vi "Create CI Frequency Channel Wrapper.vi"(0 "Task map in":map{string, refnum<k21>}(c390), 5 "Message Data in":T2, 11 "error in (no error)":errorcluster) -> (4 "Task map out":map{string, refnum<k21>}(c390), 6 "Message Data out":T1, 15 "error out":errorcluster)   [LabVIEW 2021, in "NI DAQmx_wrapper.lvlib"]
uses:
  NI DAQmx_wrapper.lvlib
  NI DAQmx_server/RPC Messages/nidaqmx_grpc_CreateCIFreqChanRequest.ctl
  NI DAQmx_server/RPC Messages/nidevice_grpc_Session_session/nidevice_grpc_Session_session.lvclass
  NI DAQmx_server/RPC Messages/nidaqmx_grpc_CreateCIFreqChanRequest_units_enum/nidaqmx_grpc_CreateCIFreqChanRequest_units_enum.lvclass
  NI DAQmx_server/RPC Messages/nidaqmx_grpc_CreateCIFreqChanRequest_edge_enum/nidaqmx_grpc_CreateCIFreqChanRequest_edge_enum.lvclass
  NI DAQmx_server/RPC Messages/nidaqmx_grpc_CreateCIFreqChanRequest_meas_method_enum/nidaqmx_grpc_CreateCIFreqChanRequest_meas_method_enum.lvclass
  NI DAQmx_server/RPC Messages/nidevice_grpc_Session.ctl
  NI DAQmx_server/RPC Messages/nidaqmx_grpc_CreateCIFreqChanResponse.ctl
  NI DAQmx_server/RPC Messages/nidaqmx_grpc_CreateCIFreqChanRequest_edge_enum/nidaqmx_grpc_CreateCIFreqChanRequest_edge_enum.lvclass/nidaqmx_grpc_CreateCIFreqChanRequest_edge_enum.ctl
  NI DAQmx_server/RPC Messages/nidaqmx_grpc_CreateCIFreqChanRequest_units_enum/nidaqmx_grpc_CreateCIFreqChanRequest_units_enum.lvclass/nidaqmx_grpc_CreateCIFreqChanRequest_units_enum.ctl
  NI DAQmx_server/RPC Messages/nidaqmx_grpc_CreateCIFreqChanRequest_meas_method_enum/nidaqmx_grpc_CreateCIFreqChanRequest_meas_method_enum.lvclass/nidaqmx_grpc_CreateCIFreqChanRequest_meas_method_enum.ctl
  NI DAQmx_server/RPC Messages/nidevice_grpc_Session_session/nidevice_grpc_Session_session.lvclass/nidevice_grpc_Session_session.ctl
  <vilib>/DAQmx/create/channels.llb/DAQmx Create Channel (CI-Frequency).vi
  NI DAQmx_server/NI DAQmx_server.lvlib
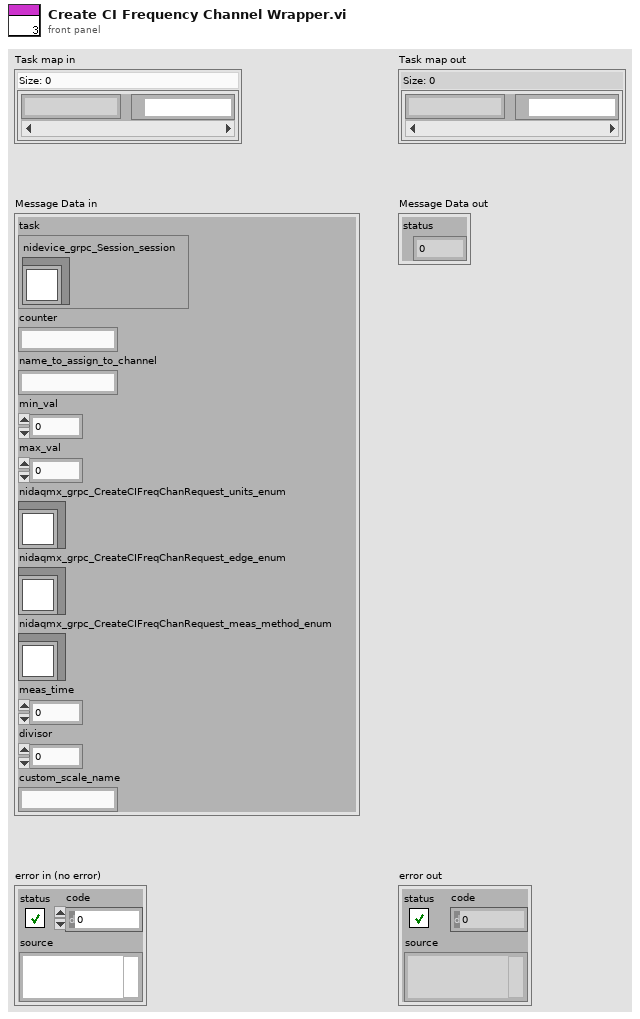
[diagram p1: front panel]
types:
  T1 = typedef "NI DAQmx_server.lvlib/nidaqmx_grpc_CreateCIFreqChanResponse.ctl" = cluster{"status":i32}
  T2 = typedef "NI DAQmx_server.lvlib/nidaqmx_grpc_CreateCIFreqChanRequest.ctl" = cluster{"task":T3, "counter":string, "name_to_assign_to_channel":string, "min_val":dbl, "max_val":dbl, "nidaqmx_grpc_CreateCIFreqChanRequest_units_enum":refnum<class "nidaqmx_grpc_CreateCIFreqChanRequest_units_enum.lvclass">, "nidaqmx_grpc_CreateCIFreqChanRequest_edge_enum":refnum<class "nidaqmx_grpc_CreateCIFreqChanRequest_edge_enum.lvclass">, "nidaqmx_grpc_CreateCIFreqChanRequest_meas_method_enum":refnum<class "nidaqmx_grpc_CreateCIFreqChanRequest_meas_method_enum.lvclass">, "meas_time":dbl, "divisor":u32, "custom_scale_name":string}
  T3 = typedef "NI DAQmx_server.lvlib/nidevice_grpc_Session.ctl" = cluster{"nidevice_grpc_Session_session":refnum<class "nidevice_grpc_Session_session.lvclass">}
  T4 = typedef "NI DAQmx_server.lvlib/nidaqmx_grpc_Edge1.ctl" = enum32{"EDGE1_UNSPECIFIED", "EDGE1_RISING", "EDGE1_FALLING"}
  T5 = typedef "NI DAQmx_server.lvlib/nidaqmx_grpc_FrequencyUnits3.ctl" = enum32{"FREQUENCY_UNITS3_UNSPECIFIED", "FREQUENCY_UNITS3_HZ", "FREQUENCY_UNITS3_TICKS", "FREQUENCY_UNITS3_FROM_CUSTOM_SCALE"}
  T6 = typedef "NI DAQmx_server.lvlib/nidaqmx_grpc_CounterFrequencyMethod.ctl" = enum32{"COUNTER_FREQUENCY_METHOD_UNSPECIFIED", "COUNTER_FREQUENCY_METHOD_LOW_FREQ_1_CTR", "COUNTER_FREQUENCY_METHOD_HIGH_FREQ_2_CTR", "COUNTER_FREQUENCY_METHOD_LARGE_RNG_2_CTR", "COUNTER_FREQUENCY_METHOD_DYN_AVG"}
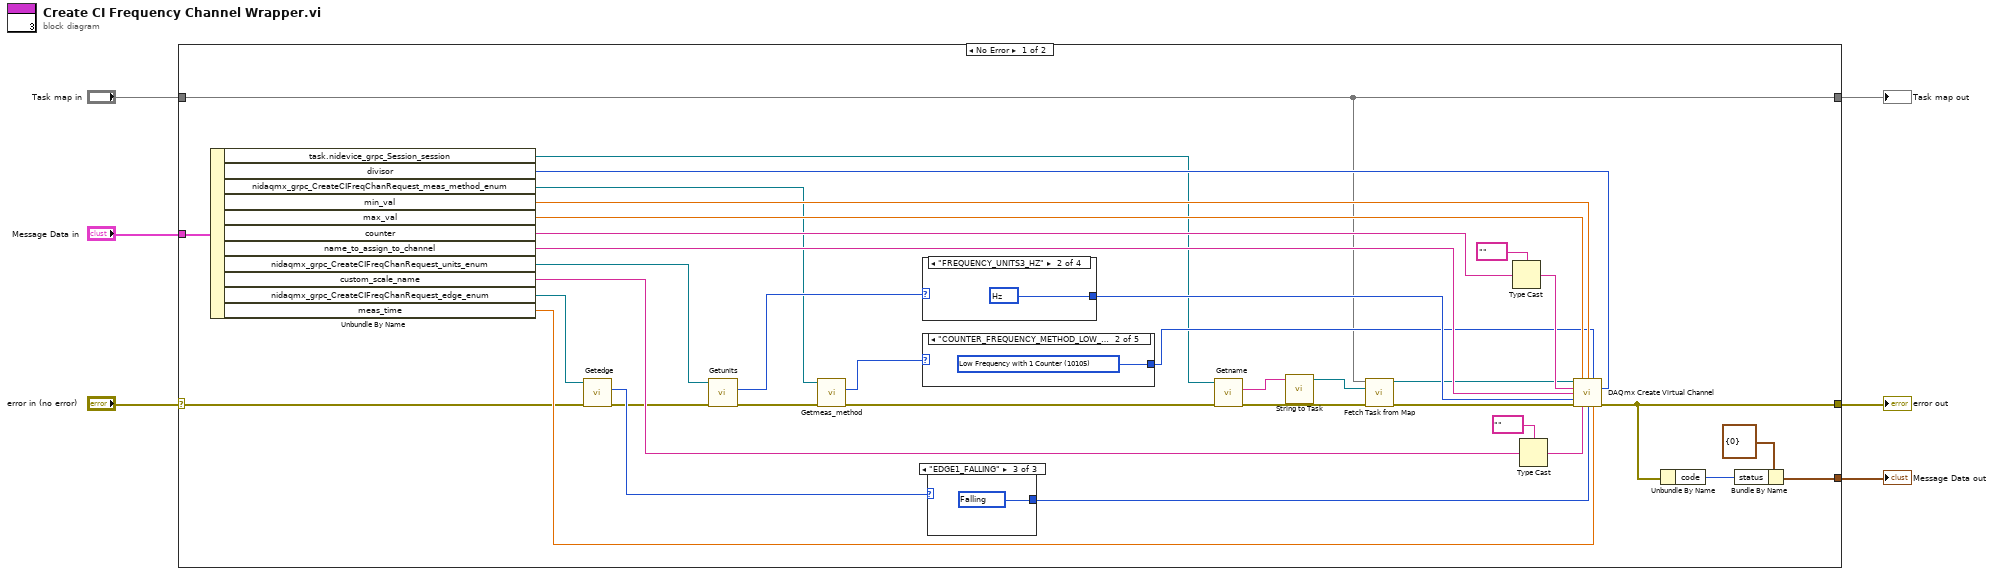
[diagram p0: block diagram]
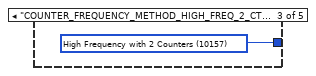
[diagram p3: hidden frame]
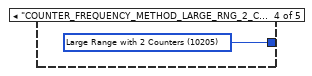
[diagram p4: hidden frame]
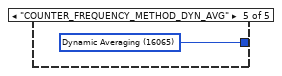
[diagram p5: hidden frame]
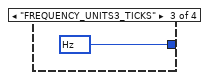
[diagram p7: hidden frame]
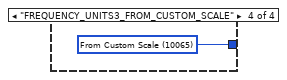
[diagram p8: hidden frame]
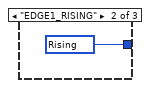
[diagram p10: hidden frame]
diagram:
  n1 = case shown="No Error" "error in (no error)" {
    selector: "error in (no error)" -> [w38 w53]
    tunnel: [w10 w53] -> w5
    tunnel: "Task map in" -> [w11 w52]
    tunnel: [w11 w52] -> w3
    tunnel: "Message Data in" -> [w42 _]
    tunnel: [w7 _] -> w1
    frame No Error {
      n2 = Unbundle By Name(w42) -> ("task.nidevice_grpc_Session_session"=w13:refnum<class "nidevice_grpc_Session_session.lvclass">, "divisor"=w23:u32, "nidaqmx_grpc_CreateCIFreqChanRequest_meas_method_enum"=w21:refnum<class "nidaqmx_grpc_CreateCIFreqChanRequest_meas_method_enum.lvclass">, "min_val"=w24:dbl, "max_val"=w25:dbl, "counter"=w26:string, "name_to_assign_to_channel"=w31:string, "nidaqmx_grpc_CreateCIFreqChanRequest_units_enum"=w29:refnum<class "nidaqmx_grpc_CreateCIFreqChanRequest_units_enum.lvclass">, "custom_scale_name"=w33:string, "nidaqmx_grpc_CreateCIFreqChanRequest_edge_enum"=w37:refnum<class "nidaqmx_grpc_CreateCIFreqChanRequest_edge_enum.lvclass">, "meas_time"=w39:dbl)
      n3 = call "Getedge.vi"("error in (no error)"=w38, "OneOfTemplate in"=w37) -> ("error out"=w30:errorcluster, "Get_Val"=w36:T4)  [unwired: 7 in, 1 out]
      n4 = call "Getunits.vi"("error in (no error)"=w30, "OneOfTemplate in"=w29) -> ("error out"=w22:errorcluster, "Get_Val"=w28:T5)  [unwired: 7 in, 1 out]
      n5 = call "Getmeas_method.vi"("error in (no error)"=w22, "OneOfTemplate in"=w21) -> ("error out"=w15:errorcluster, "Get_Val"=w20:T6)  [unwired: 7 in, 1 out]
      n6 = case shown="\"FREQUENCY_UNITS3_HZ\"" w28 {
        tunnel: [_ w47 w48 w49] -> w27
        frame "FREQUENCY_UNITS3_UNSPECIFIED", Default {
        }
        frame "FREQUENCY_UNITS3_HZ" {
          w47 = 10373 items=["Hz"=10373, "Ticks"=10304, "From Custom Scale"=10065] ("units")
        }
        frame "FREQUENCY_UNITS3_TICKS" {
          w48 = 10373 items=["Hz"=10373, "Ticks"=10304, "From Custom Scale"=10065] ("units")
        }
        frame "FREQUENCY_UNITS3_FROM_CUSTOM_SCALE" {
          w49 = 10065 items=["Hz"=10373, "Ticks"=10304, "From Custom Scale"=10065] ("units")
        }
      }
      n7 = case shown="\"COUNTER_FREQUENCY_METHOD_LOW_FREQ_1_CTR\"" w20 {
        tunnel: [_ w43 w44 w45 w46] -> w19
        frame "COUNTER_FREQUENCY_METHOD_UNSPECIFIED", Default {
        }
        frame "COUNTER_FREQUENCY_METHOD_LOW_FREQ_1_CTR" {
          w43 = 10105 items=["Low Frequency with 1 Counter"=10105, "High Frequency with 2 Counters"=10157, "Large Range with 2 Counters"=10205, "Dynamic Averaging"=16065] ("measurement method")
        }
        frame "COUNTER_FREQUENCY_METHOD_HIGH_FREQ_2_CTR" {
          w44 = 10157 items=["Low Frequency with 1 Counter"=10105, "High Frequency with 2 Counters"=10157, "Large Range with 2 Counters"=10205, "Dynamic Averaging"=16065] ("measurement method")
        }
        frame "COUNTER_FREQUENCY_METHOD_LARGE_RNG_2_CTR" {
          w45 = 10205 items=["Low Frequency with 1 Counter"=10105, "High Frequency with 2 Counters"=10157, "Large Range with 2 Counters"=10205, "Dynamic Averaging"=16065] ("measurement method")
        }
        frame "COUNTER_FREQUENCY_METHOD_DYN_AVG" {
          w46 = 16065 items=["Low Frequency with 1 Counter"=10105, "High Frequency with 2 Counters"=10157, "Large Range with 2 Counters"=10205, "Dynamic Averaging"=16065] ("measurement method")
        }
      }
      n8 = case shown="\"EDGE1_FALLING\"" w36 {
        tunnel: [_ w50 w51] -> w35
        frame "EDGE1_UNSPECIFIED", Default {
        }
        frame "EDGE1_RISING" {
          w50 = 10280 items=["Rising"=10280, "Falling"=10171] ("starting edge")
        }
        frame "EDGE1_FALLING" {
          w51 = 10171 items=["Rising"=10280, "Falling"=10171] ("starting edge")
        }
      }
      n9 = call "Getname.vi"("error in (no error)"=w15, "OneOfTemplate in"=w13) -> ("error out"=w17:errorcluster, "Get_Val"=w18:string)  [unwired: 7 in, 1 out]
      n10 = call "String to Task.vi"("Get_Val"=w18) -> ("Refnum out"=w16:refnum<k21>)  [unwired: 10 in]
      n11 = call "Fetch Task from Map.vi"("Task map in"=w11, "Task in"=w16, "error in (no error)"=w17) -> ("Task out"=w12:refnum<k21>, "error out"=w14:errorcluster)  [unwired: 11 in]
      n12 = Type Cast(type=tag "" ("counter"), x=w26) -> (*(type *) &x=w40:tag)
      n13 = Type Cast(type=tag "" ("custom scale name"), x=w33) -> (*(type *) &x=w32:tag)
      n14 = call-poly <vilib>:"DAQmx Create Virtual Channel.vi"("task in"=w12, "maximum value"=w25, "minimum value"=w24, "measurement method"=w19, "counter"=w40, "divisor"=w23, "name to assign"=w31, "units"=w27, "error in"=w14, "custom scale name"=w32, "starting edge"=w35, "measurement time"=w39) -> ("error out"=w10:errorcluster)  [unwired: 2 in, 1 out]
      n15 = Unbundle By Name(w10) -> ("code"=w8:i32)
      n16 = Bundle By Name(cluster=T1 {"status"=0} ("Message Data"), "status"=w8) -> (w7:T1)
    }
    frame Error {
    }
  }
  "error out" <- w5
  "Task map out" <- w3
  "Message Data out" <- w1
